vi "Append a Table of Contents.vi"(0 "PDF Report IN":refnum<class "PDF Report Class.lvclass">, 1 "Title Font":T1={"Name"="", "Size"=-1.0, "Color"=0, "Style"={"Bold"=TRUE, "Italic"=FALSE, "Underline"=FALSE, "Strikeout"=FALSE}, "Type"={"Type&direction"=enum."Select", "Embedded"=FALSE, "Encoding"=""}}, 2 "Title":string="Table of Contents", 11 "error in (no error)":errorcluster, 12 "Chapter and section Font":T1={"Name"="", "Size"=-1.0, "Color"=0, "Style"={"Bold"=TRUE, "Italic"=FALSE, "Underline"=FALSE, "Strikeout"=FALSE}, "Type"={"Type&direction"=enum."Select", "Embedded"=FALSE, "Encoding"=""}}) -> (4 "PDF Report OUT":refnum<class "PDF Report Class.lvclass">, 15 "error out":errorcluster)   [LabVIEW 2020, in "Exaprom PDF.lvlib"]
doc: "Version 1.1\nDeveloped by Jean-Marc Simard\nCopyright © 2012, Exaprom Inc.\nAll rights reserved.\nLicense: BSD\n\nWith iTextSharp 4.1.6 (http://itextsharp.sourceforge.net)\nunder Mozilla Public License Version 1.1\n(http://www.mozilla.org/MPL/MPL-1.1.html)"
uses:
  <userlib>/labview-PDF-writer-master/Exaprom PDF.lvlib
  <userlib>/labview-PDF-writer-master/LV Class/PDF Report Class/PDF Report Class.lvclass
  <userlib>/labview-PDF-writer-master/Controls/Font Controls/Font complete cluster.ctl
  <userlib>/labview-PDF-writer-master/Controls/Font Controls/Font size.ctl
  <userlib>/labview-PDF-writer-master/Controls/Font Controls/Font color.ctl
  <userlib>/labview-PDF-writer-master/Controls/Font Controls/Type and encoding.ctl
  <userlib>/labview-PDF-writer-master/Controls/Text Controls/Unicode/Type and run direction.ctl
  C:/Program Files (x86)/National Instruments/LabVIEW 2020/user.lib/labview-PDF-writer-master/DLL/itextsharp.dll
  DLL/itextsharp.dll
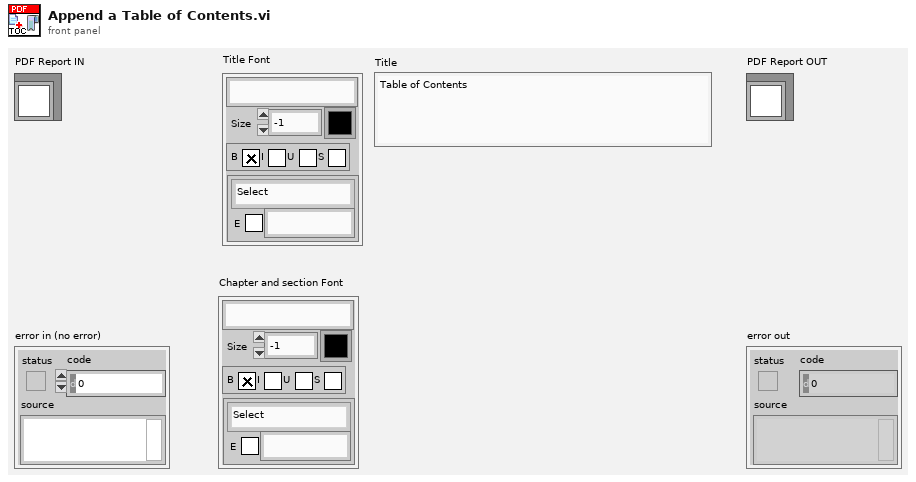
[diagram p1: front panel]
types:
  T1 = typedef "Exaprom PDF.lvlib/Font complete cluster.ctl" = cluster{"Name":string, "Size":T2, "Color":T3, "Style":cluster{"Bold":bool, "Italic":bool, "Underline":bool, "Strikeout":bool}, "Type":T4}
  T2 = typedef "Exaprom PDF.lvlib/Font size.ctl" = sgl
  T3 = typedef "Exaprom PDF.lvlib/Font color.ctl" = u32
  T4 = typedef "Exaprom PDF.lvlib/Type and encoding.ctl" = cluster{"Type&direction":T5, "Embedded":bool, "Encoding":string}
  T5 = typedef "Exaprom PDF.lvlib/Type and run direction.ctl" = enum16{"Select", "ASCII", "UTF-16", "UTF-16 (default)", "UTF-16 (LTR)", "UTF-16 (RTL)"}
  T6 = cluster{"Title":string, "Title Font":T1, "Chapter and section Font":T1, i32, "Add TOC?":bool}
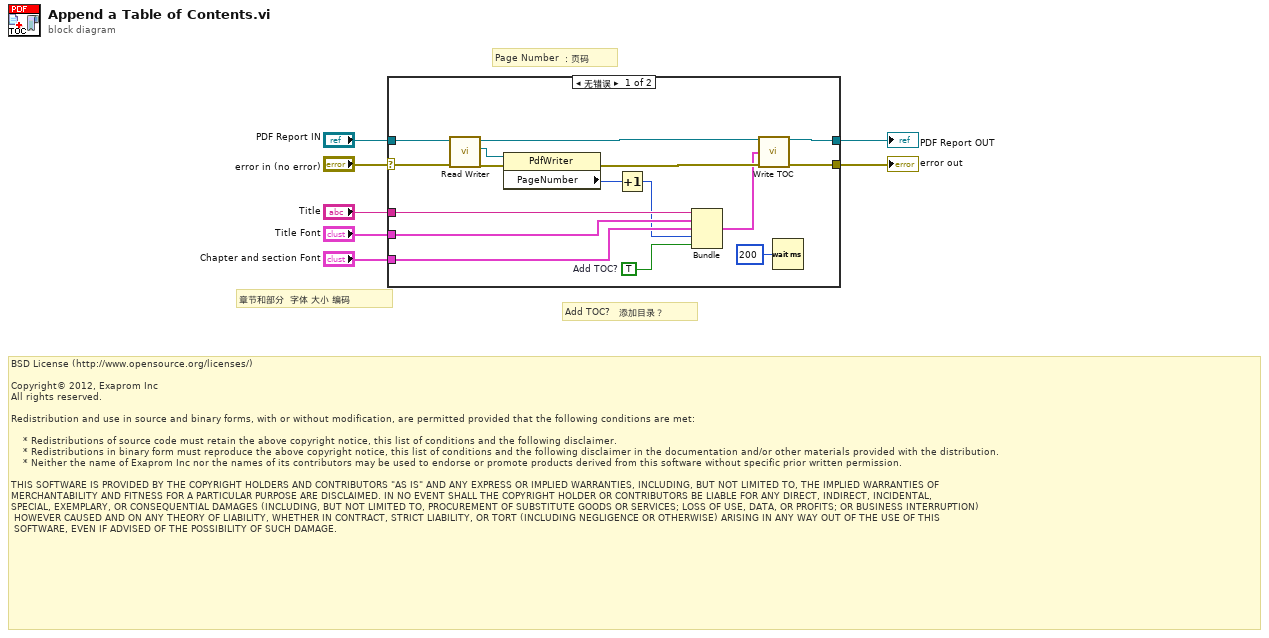
[diagram p0: block diagram]
diagram:
  # "章节和部分  字体 大小 编码"
  # "Page Number ：页码"
  # "Add TOC?   添加目录？"
  # "BSD License (http://www.opensource.org/licenses/)\n\nCopyright© 2012, Exaprom Inc\nAll rights reserved.\n\nRedistribution and use in source and binary forms, with or without modification, are permitted provided that the following conditions are met:\n\n    * Redistributions of source code must retain the above copyright notice, this list of conditions and the following disclaimer.\n    * Redistributions in binary form must reproduce the above copyright notice, this list of conditions and the following disclaimer in the documentation and/or other materials provided with the distribution.\n    * Neither the name of Exaprom Inc nor the names of its contributors may be used to endorse or promote products derived from this software without specific prior written permission.\n\nTHIS SOFTWARE IS PROVIDED BY THE COPYRIGHT HOLDERS AND CONTRIBUTORS \"AS IS\" AND ANY EXPRESS OR IMPLIED WARRANTIES, INCLUDING, BUT NOT LIMITED TO, THE IMPLIED WARRANTIES OF \nMERCHANTABILITY AND FITNESS FOR A PARTICULAR PURPOSE ARE DISCLAIMED. IN NO EVENT SHALL THE COPYRIGHT HOLDER OR CONTRIBUTORS BE LIABLE FOR ANY DIRECT, INDIRECT, INCIDENTAL,\nSPECIAL, EXEMPLARY, OR CONSEQUENTIAL DAMAGES (INCLUDING, BUT NOT LIMITED TO, PROCUREMENT OF SUBSTITUTE GOODS OR SERVICES; LOSS OF USE, DATA, OR PROFITS; OR BUSINESS INTERRUPTION)\n HOWEVER CAUSED AND ON ANY THEORY OF LIABILITY, WHETHER IN CONTRACT, STRICT LIABILITY, OR TORT (INCLUDING NEGLIGENCE OR OTHERWISE) ARISING IN ANY WAY OUT OF THE USE OF THIS\n SOFTWARE, EVEN IF ADVISED OF THE POSSIBILITY OF SUCH DAMAGE."
  n1 = case shown="无错误" "error in (no error)" {
    selector: "error in (no error)" -> [w20 w24]
    tunnel: "PDF Report IN" -> [w23 w25]
    tunnel: [w21 w25] -> w6
    tunnel: [w18 w24] -> w5
    tunnel: "Title" -> [w14 _]
    tunnel: "Title Font" -> [w13 _]
    tunnel: "Chapter and section Font" -> [w12 _]
    frame No Error {
      w10 = TRUE  # Add TOC?
      n2 = call-dynamic "Read Writer.vi"("error in (no error)"=w20, "PDF Report Class in"=w23) -> ("error out"=w19:errorcluster, "Writer"=w16:refnum<k24>, "PDF Report Class out"=w22:refnum<class "PDF Report Class.lvclass">)  [unwired: 7 in]
      n3 = property class="PdfWriter"(reference=w16, error in=w19) -> (error out=w17:errorcluster, "PageNumber"=w11:i32)  [unwired: 1 out]
      n4 = Increment(x=w11) -> (x+1=w9:i32)
      n5 = Bundle("Title"=w14, "Title Font"=w13, "Chapter and section Font"=w12, w9, "Add TOC?"=w10) -> (w15:T6)  [unwired: 1 in]
      n6 = call-dynamic "Write TOC.vi"("PDF Report Class in"=w22, "TOC"=w15, "error in (no error)"=w17) -> ("PDF Report Class out"=w21:refnum<class "PDF Report Class.lvclass">, "error out"=w18:errorcluster)  [unwired: 11 in]
      n7 = Wait (ms)(milliseconds to wait=u32 200 ("等待时间（毫秒）")) -> ()  [unwired: 1 out]
    }
    frame Error {
    }
  }
  "PDF Report OUT" <- w6
  "error out" <- w5
